vi "Write to StdOut of Calling Parent.vi"(4 "error in":errorcluster, 7 "StdOut":string) -> (0 "error out":errorcluster)   [LabVIEW 2018]
doc: "This VI is used to send text output to the StdOut of the console app that calls the executable build with this VI. This is accomplised with calls to the Windows kernel32.dll."
uses:
  kernel32.dll
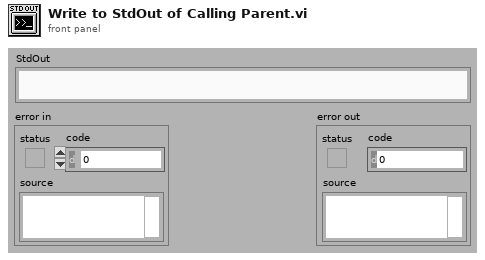
[diagram p1: front panel]
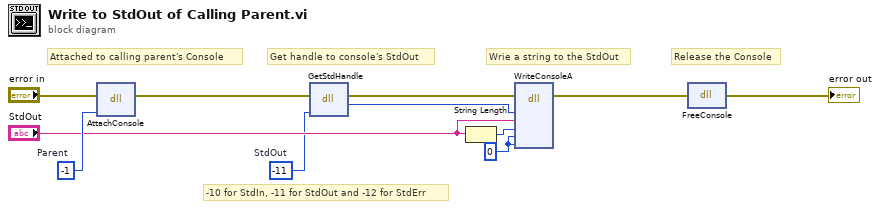
[diagram p0: block diagram]
diagram:
  w9 = -1  # Parent
  w4 = -11  # StdOut
  w6 = 0 ("lpNumberOfCharsWritten")
  # "Release the Console"
  # "Wrie a string to the StdOut"
  # "Get handle to console's StdOut"
  # "Attached to calling parent's Console"
  # "-10 for StdIn, -11 for StdOut and -12 for StdErr"
  n1 = dll-call lib="kernel32.dll" fn="AttachConsole"(error in="error in", "arg1"=w9) -> (error out=w10:errorcluster)  [unwired: 3 in, 2 out]
  n2 = dll-call lib="kernel32.dll" fn="GetStdHandle"(error in=w10, "nStdHandle"=w4) -> (error out=w3:errorcluster, "return type"=w5:i32)  [unwired: 3 in, 1 out]
  n3 = String Length(string="StdOut") -> (length=w7:i32)
  n4 = dll-call lib="kernel32.dll" fn="WriteConsoleA"(error in=w3, "hConsoleOutput"=w5, "lpBuffer"="StdOut", "numberOfCharsToWrite"=w7, "lpNumberOfCharsWritten"=w6, "lpReserved"=w6) -> (error out=w2:errorcluster)  [unwired: 5 in, 4 out]
  n5 = dll-call lib="kernel32.dll" fn="FreeConsole"(error in=w2) -> (error out=→"error out":errorcluster)  [unwired: 2 in, 2 out]
